vi "Drive Motor Init.vi"(11 "Error In":errorcluster) -> (2 "Drive Motor Handle":T1, 3 "Error Out":errorcluster)   [LabVIEW 2021]
uses:
  Drive Motor Handle.ctl
  <vilib>/Instr/_visa.llb/VISA Configure Serial Port (Instr).vi
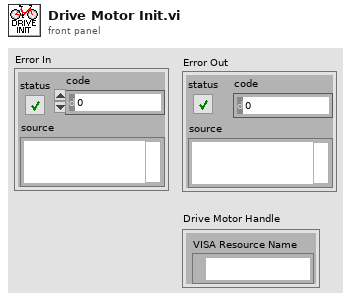
[diagram p1: front panel]
types:
  T1 = typedef "Drive Motor Handle.ctl" = cluster{"VISA Resource Name":refnum<visa-resource-name>}
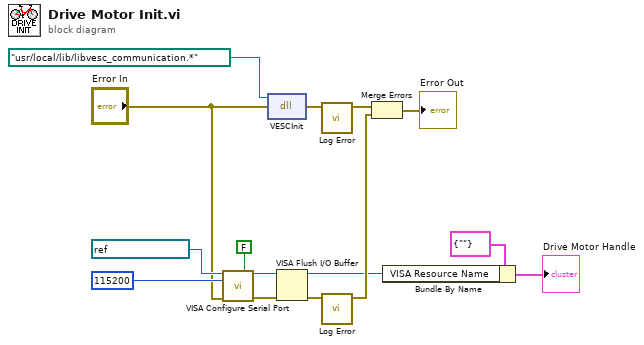
[diagram p0: block diagram]
diagram:
  n1 = call-poly "VISA Configure Serial Port"("VISA resource name"=refnum<visa-resource-name> "ASRL2::INSTR", "Enable Termination\nChar (T)"=FALSE ("Enable Termination\nChar (T)"), "baud rate (9600)"=u32 115200, "error in (no error)"="Error In") -> ("VISA resource name out"=w2:refnum<visa-resource-name>, "error out"=w1:errorcluster)  [unwired: 10 in]
  n2 = dll-call lib="?" fn="VESCInit"(path in=path "/usr/local/lib/libvesc_communication.*", error in="Error In") -> (error out=w14:errorcluster)  [unwired: 2 in, 1 out]
  n3 = VISA Flush I/O Buffer(VISA resource name=w2, error in (no error)=w1) -> (VISA resource name out=w3:refnum<visa-resource-name>, error out=w5:errorcluster)  [unwired: 1 in]
  n4 = call "Log Error.vi"("Error In"=w14) -> ("Error Out"=w7:errorcluster)  [unwired: 10 in]
  n5 = call "Log Error.vi"("Error In"=w5) -> ("Error Out"=w4:errorcluster)  [unwired: 10 in]
  n6 = Merge Errors(w7, w4) -> (→"Error Out":errorcluster)
  n7 = Bundle By Name(cluster=T1 {"VISA Resource Name"=""} ("Drive Motor Handle"), "VISA Resource Name"=w3) -> (→"Drive Motor Handle":T1)
